vi "4.3-How.vi"() -> ()   [LabVIEW 2010]
uses:
  2-Low Neurons/2.4-How Sensor Typedef.ctl
  <vilib>/Platform/TimedLoop/XDataNode/XDataNode.xnode
  <vilib>/Platform/TimedLoop/XDataNode/timing_clust.ctl
  <vilib>/Platform/TimedLoop/XDataNode/nitl_modes.ctl
  <vilib>/Platform/TimedLoop/XDataNode/wakeup.ctl
  <vilib>/rvi/interface/nirviReadWriteControl/nirviReadWriteControl.xnode
  4-High Neurons/4.1-FPGA VI Typedef.ctl
  FPGA Bitfiles/DaveBrain_FPGATarget_1-Hindbrain2_BC392278.lvbitx
  1-Hindbrain.vi
  <vilib>/rvi/interface/common/niFpgaNodeNameForErrorReporting.ctl
  <vilib>/rvi/errors/niLvFpgaWhatHappensToTopLevelVI.ctl
  3.0-Global.vi
  <vilib>/Utility/error.llb/Error Cluster From Error Code.vi
  <vilib>/rvi/errors/niLvFpgaAdjustHostInterfaceError.vi
  <vilib>/Platform/TimedLoop/XDataNode/XDNodeRunTimeDep.lvlib
  NiFpgaLv.dll
panel:
  out "2.4 How Am I? Sensor":T1
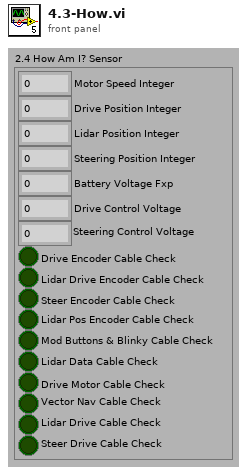
[diagram p1: front panel]
types:
  T1 = typedef "2.4-How Sensor Typedef.ctl" = cluster{"Motor Speed Integer":i16, "Drive Position Integer":i32, "Lidar Position Integer":i32, "Steering Position Integer":i32, "Battery Voltage Fxp":fxp<+/-,16,5>, "Drive Control Voltage":fxp<+/-,20,5>, "Steering Control Voltage":fxp<+/-,20,5>, "Drive Encoder Cable Check":bool, "Lidar Drive Encoder Cable Check":bool, "Steer Encoder Cable Check":bool, "Lidar Pos Encoder Cable Check":bool, "Mod Buttons & Blinky Cable Check":bool, "Lidar Data Cable Check":bool, "Drive Motor Cable Check":bool, "Vector Nav Cable Check":bool, "Lidar Drive Cable Check":bool, "Steer Drive Cable Check":bool}
  T2 = typedef "XDNodeRunTimeDep.lvlib/timing_clust.ctl" = cluster{"Expected End [f-1]":u64, "Actual End [f-1]":u64, "Finished Late? [f-1]":bool, "Expected End [i-1]":u64, "Actual End [i-1]":u64, "Finished Late? [i-1]":bool, "Expected Start [i]":u64, "Actual Start [i]":u64, "Expected Start [f]":u64, "Actual Start [f]":u64, "Source Name":string, "Structure Name":string, "Period":i64, "Deadline":i64, "Offset":i64, "Start":i64, "Priority":i32, "Timeout":i32, "Mode":T3, "Wakeup Reason":T4, "Error":errorcluster, "Source Type":string, "Secondary Source Type":string, "Global End Time":u64, "Global Start Time":u64, "Frame Duration":u64, "Iteration Duration":u64, "Assigned CPU":i32, "I/O Scan Engine Mode":u32}
  T3 = typedef "XDNodeRunTimeDep.lvlib/nitl_modes.ctl" = enum32{"No Change", "Process missed periods, maintain original phase", "Discard missed periods, maintain original phase", "Process missed periods, ignore original phase", "Discard missed periods, ignore original phase"}
  T4 = typedef "XDNodeRunTimeDep.lvlib/wakeup.ctl" = enum32{"Normal", "Aborted", "Asynchronous wakeup", "Timing source error", "Timed loop error", "Timeout"}
  T5 = typedef "niFpgaNodeNameForErrorReporting.ctl" = enum16{"Open FPGA VI Reference", "Read/Write Control", "Invoke Method: Abort", "Invoke Method: Acknowledge IRQ", "Invoke Method: Download", "Invoke Method: FIFO.Configure", "Invoke Method: FIFO.Read", "Invoke Method: FIFO.Start", "Invoke Method: FIFO.Stop", "Invoke Method: FIFO.Write", "Invoke Method: Reset", "Invoke Method: Run", "Invoke Method: Wait on IRQ", "Close FPGA VI Reference"}
  T6 = typedef "niLvFpgaWhatHappensToTopLevelVI.ctl" = enum16{"top level VI scripted behind XNode", "top level VI inlined behind XNode"}
  T7 = typedef "4.1-FPGA VI Typedef.ctl" = refnum<k20>
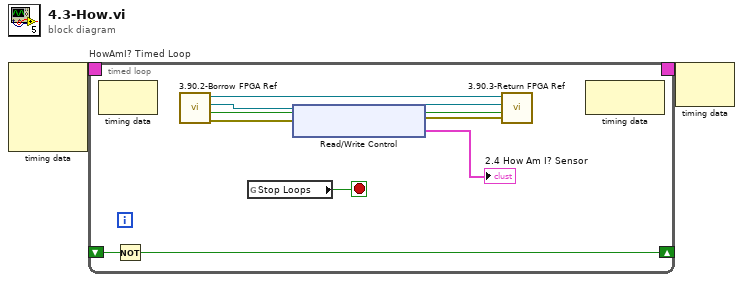
[diagram p0: block diagram]
diagram:
  n1 = node-c288 ("Input Node")() -> (w2:T2)  [unwired: 4 in]
  n2 = timed-loop "HowAmI? Timed Loop" {
    timing: w2 -> [_]
    timing-out: [_] -> w1
    shift-right: [w11] -> _
    shift-left: _ -> [w12]
    stop <- w3 stop-if-true
    n3 = node-c288() -> ()  [unwired: 1 in, 1 out]
    n4 = Not(x=w12) -> (.not. x?=w11:bool)
    n5 = call "3.90.2-Borrow FPGA Ref.vi"() -> ("error out"=w6:errorcluster, "Failed to Obtain Ref"=w10:bool, "element"=w9:T7, "FPGA Ref"=w8:refnum<queue>)  [unwired: 4 in]
    n6 = global read "3.0-Global.vi" "Stop Loops"() -> (w3:bool)
    n7 = xnode "Read/Write Control"("FPGA VI Reference In"=w9, "error in"=w6) -> ("FPGA VI Reference Out"=w7:T7, "error out"=w5:errorcluster, "2.4 How Am I? Sensor"=→"2.4 How Am I? Sensor":T1)
    n8 = call "3.90.3-Return FPGA Ref.vi"("error in"=w5, "Failed to Obtain Ref"=w10, "element"=w7, "FPGA Ref"=w8) -> ()  [unwired: 1 out]
    n9 = node-c288() -> ()  [unwired: 1 in, 1 out]
  }
  n10 = node-c288(w1) -> ()  [unwired: 1 out]
